vi "Write Drag Starting Filtered Event.vi"(6 "Drag Starting Filtered Event":refnum<notifier>, 11 "Handle Drag Starting Msg in":refnum<class "Handle Drag Starting Msg.lvclass">) -> (3 "Handle Drag Starting Msg out":refnum<class "Handle Drag Starting Msg.lvclass">)   [LabVIEW 2017, in "Handle Drag Starting Msg.lvclass"]
uses:
  <vilib>/gpm_packages/@cs/Test-executive-builder/Source/Test Executive Builder View/Test Executive Builder View Messages/Handle Drag Starting Msg/Handle Drag Starting Msg.lvclass
  <vilib>/gpm_packages/@cs/Test-executive-builder/Source/Application Dependencies/Drag Starting Filtered Event Data.ctl
  <vilib>/gpm_packages/@cs/Test-executive-builder/Source/Test Executive Builder View/Test Executive Builder View Messages/Handle Drag Starting Msg/Handle Drag Starting Msg.lvclass/Handle Drag Starting Msg.ctl
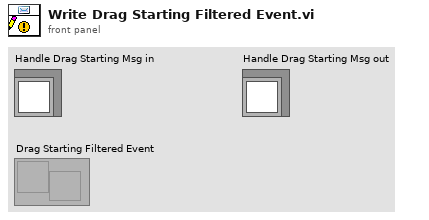
[diagram p1: front panel]
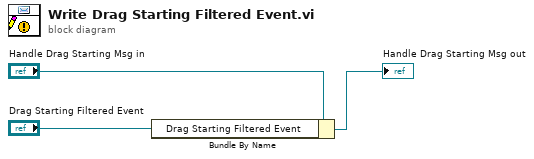
[diagram p0: block diagram]
diagram:
  n1 = Bundle By Name(cluster="Handle Drag Starting Msg in", "Drag Starting Filtered Event"="Drag Starting Filtered Event") -> (→"Handle Drag Starting Msg out":refnum<class "Handle Drag Starting Msg.lvclass">)
